vi "FGV-StatusChangeEventRef.vi"(8 "error in (no error)":errorcluster, 11 "Name(\"\" to use uuid) in":string) -> (0 "error out":errorcluster, 3 "Status Change Event":refnum<user-event>)   [LabVIEW 2014, in "JKI State Machine++.lvlib"]
uses:
  JKI State Machine++.lvlib
  Typedef/_JKISM Status Change Event Data.ctl
  JKISMQ/_JKISMQFGVOPER.ctl
  FGV-BroadcastRegistry/global-JKISMQ FGV Change Flag.vi
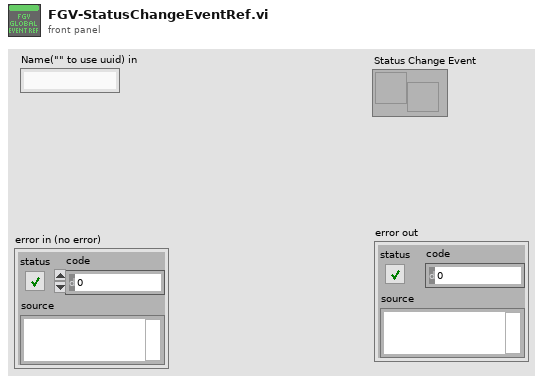
[diagram p1: front panel]
types:
  T1 = typedef "JKI State Machine++.lvlib/_JKISMQFGVOPER.ctl" = enum16{"Get By Name", "List", "Check If Name Exists", "Release", "Module Status", "Create Status Event Handler", "Destroy Status Event Handler"}
  T2 = typedef "JKI State Machine++.lvlib/_JKISMQ.ctl" = cluster{"Module Name":string, "Queue":refnum<queue>, "Locked Status":refnum<data-value>, "Mode":T3, "User Event":refnum<user-event>, "Queue Count":i32, "Status Change Event":refnum<user-event>}
  T3 = typedef "JKI State Machine++.lvlib/_JKISM_MODE.ctl" = enum16{"Stand Alone", "JKISM", "Action Worker"}
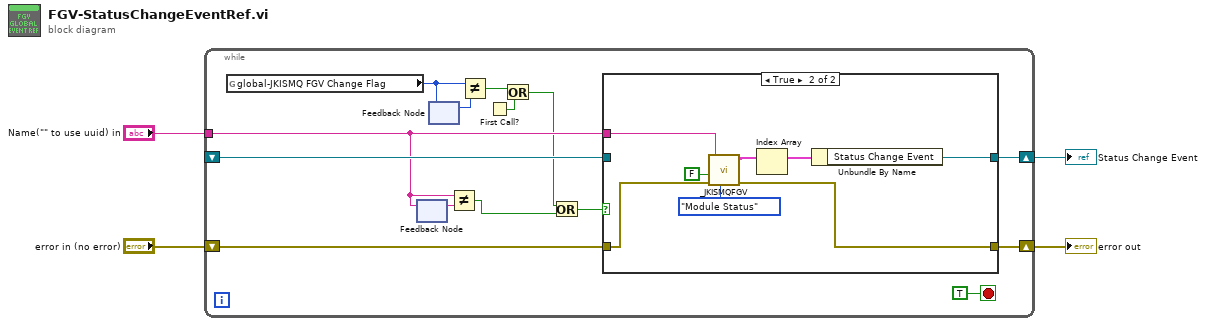
[diagram p0: block diagram]
diagram:
  n1 = while {
    shift-right: [w16] -> w2
    shift-left: "error in (no error)" -> [w17]
    shift-right: [w18] -> w4
    shift-left: _ -> [w14]
    tunnel: "Name(\"\" to use uuid) in" -> [w13]
    stop <- TRUE stop-if-true
    n2 = global read "global-JKISMQ FGV Change Flag.vi" "global-JKISMQ FGV Change Flag"() -> (w10:u32)
    n3 = feedback-in #1(w13) -> ()
    n4 = feedback #1() -> (w12:string)  [unwired: 1 in]
    n5 = feedback #2() -> (w9:u32)  [unwired: 1 in]
    n6 = feedback-in #2(w10) -> ()
    n7 = Not Equal?(x=w13, y=w12) -> (x != y?=w11:bool)
    n8 = Not Equal?(x=w10, y=w9) -> (x != y?=w7:bool)
    n9 = First Call?() -> (First Call?: T/F=w8:bool)
    n10 = Or(x=w7, y=w8) -> (x .or. y?=w6:bool)
    n11 = Or(x=w6, y=w11) -> (x .or. y?=w5:bool)
    n12 = case shown="True" w5 {
      tunnel: [w20 w23] -> w18
      tunnel: w17 -> [w19 w26]
      tunnel: [w19 w27] -> w16
      tunnel: w14 -> [w20 _]
      tunnel: w13 -> [_ w22]
      frame False {
      }
      frame True {
        n13 = call "_JKISMQFGV.vi"("Operation"=_JKISMQFGVOPER."Module Status", "Error in"=w26, "create if not found? (T)"=FALSE, "Name(\"\" to use uuid) in"=w22) -> ("Error out"=w27:errorcluster, "Array"=w25:T2[])  [unwired: 4 in, 2 out]
        n14 = Index Array(array=w25) -> (element=w24:T2)  [unwired: 1 in]
        n15 = Unbundle By Name(w24) -> ("Status Change Event"=w23:refnum<user-event>)
      }
    }
  }
  "Status Change Event" <- w4
  "error out" <- w2
